vi "initialize Session Data.vi"(0 "OBJ - Session in":refnum<class "FPGA Serial Session.lvclass">, 11 "error in":errorcluster) -> (4 "OBJ - Session out":refnum<class "FPGA Serial Session.lvclass">, 15 "error out":errorcluster)   [LabVIEW 2015, in "FPGA Serial Session.lvclass"]
doc: "OVERRIDE VI\nPlaceholder for decendant sessions to initialize and set their default values"
uses:
  FPGA Serial Session.lvclass
  Reusable/Session APIs/File Access/Config Data/Config Data.lvclass
  Reusable/Session APIs/File Access/Config Data/Config Data.lvclass/Config Data.ctl
  FPGA Serial Session.lvclass/FPGA Serial Session.ctl
  Reusable/Session APIs/File Access/Config Data/Accessors/Read Ref.vi
  <vilib>/Utility/config.llb/Read Key (String).vi
  <vilib>/Utility/config.llb/Read Key (I32).vi
  <userlib>/_Session Fwk/Session - Root.lvclass
  Reusable/Session APIs/Text Communication/Text Device Session.lvclass
  <vilib>/Utility/config.llb/NI_LVConfig.lvlib
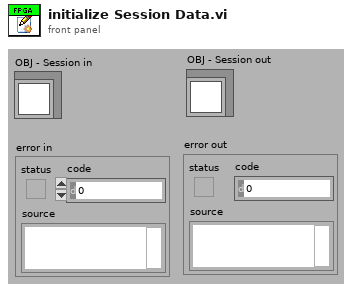
[diagram p1: front panel]
types:
  T1 = typedef "Session - Root.lvclass/Session Handle.ctl" = refnum<data-value>
  T2 = typedef "NI_LVConfig.lvlib/Config Data RefNum.ctl" = refnum<k1>
  T3 = enum16{"Port 1", "Port 2", "Port 3", "Port 4", "None"}
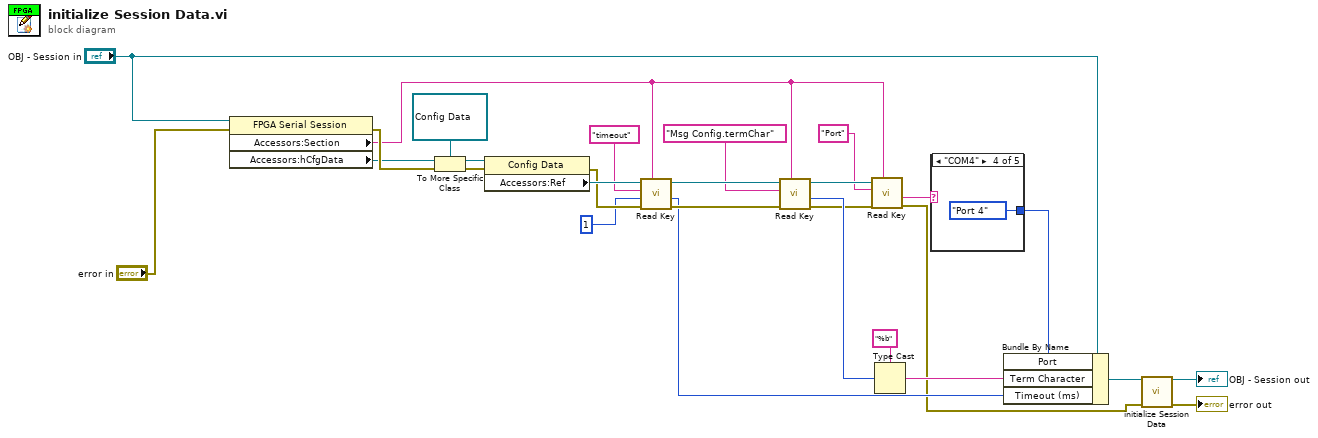
[diagram p0: block diagram]
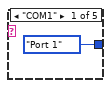
[diagram p2: hidden frame]
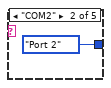
[diagram p3: hidden frame]
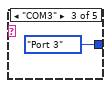
[diagram p4: hidden frame]
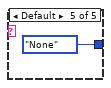
[diagram p5: hidden frame]
diagram:
  n1 = property class="FPGA Serial Session"(reference="OBJ - Session in", error in="error in") -> (error out=w25:errorcluster, "Accessors:Section"=w9:string, "Accessors:hCfgData"=w23:T1)  [unwired: 1 out]
  n2 = To More Specific Class(target class=refnum<data-value> refnum, reference=w23, error in=w25) -> (specific class reference=w27:refnum<data-value>, error out=w26:errorcluster)
  n3 = property class="Config Data"(reference=w27, error in=w26) -> (error out=w21:errorcluster, "Accessors:Ref"=w24:T2)  [unwired: 1 out]
  n4 = call-poly <vilib>:"Read Key.vi"("section"=w9, "error in (no error)"=w21, "default value"=1, "key"="timeout", "refnum"=w24) -> ("error out"=w19:errorcluster, "value"=w13:i32, "refnum out"=w20:T2)  [unwired: 3 in, 1 out]
  n5 = call-poly <vilib>:"Read Key.vi"("section"=w9, "error in (no error)"=w19, "key"="Msg Config.termChar", "refnum"=w20) -> ("error out"=w11:errorcluster, "value"=w16:i32, "refnum out"=w12:T2)  [unwired: 4 in, 1 out]
  n6 = call-poly <vilib>:"Read Key.vi"("section"=w9, "error in (no error)"=w11, "key"="Port", "refnum"=w12) -> ("error out"=w3:errorcluster, "value"=w8:string)  [unwired: 4 in, 2 out]
  n7 = Type Cast(type="%b", x=w16) -> (*(type *) &x=w14:string)
  n8 = case shown="\"COM4\"" w8 {
    tunnel: [T3."Port 1" ("Port") T3."Port 2" ("Port") T3."Port 3" ("Port") T3."Port 4" ("Port") T3."None" ("Port")] -> w7
    frame "COM1" {
    }
    frame "COM2" {
    }
    frame "COM3" {
    }
    frame "COM4" {
    }
    frame Default {
    }
  }
  n9 = Bundle By Name(cluster="OBJ - Session in", "Port"=w7, "Term Character"=w14, "Timeout (ms)"=w13) -> (w5:refnum<class "FPGA Serial Session.lvclass">)
  n10 = call-parent "initialize Session Data.vi"("OBJ - Session in"=w5, "error in"=w3) -> ("OBJ - Session out"=→"OBJ - Session out":refnum<class "FPGA Serial Session.lvclass">, "error out"=→"error out":errorcluster)  [unwired: 12 in]
